vi "Close.vi"(8 "error in (no error)":errorcluster, 11 "reference in":refnum<class "Test_Sim.lvclass">) -> (0 "error out":errorcluster, 3 "reference in":refnum<class "Test_Sim.lvclass">)   [LabVIEW 2020, in "Test_Sim.lvlib" / "Test_Sim.lvclass"]
uses:
  Test_Sim.lvclass
  Components/Test_Base.lvlibp/Test_Base.lvclass
  Components/ViPER.lvlibp/ViPER.lvclass
  C:/Projects/Medulla/Presentations/Sydney_LVUG/Demo/Flux_Capacitor_Tester/Components/ViPER.lvlibp/ViPER.lvclass
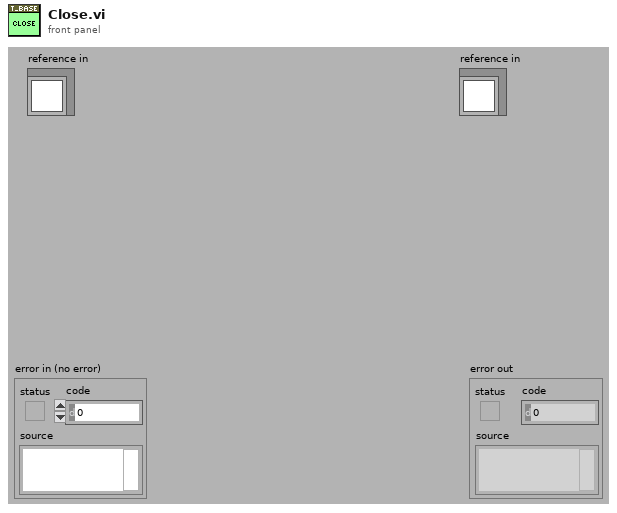
[diagram p1: front panel]
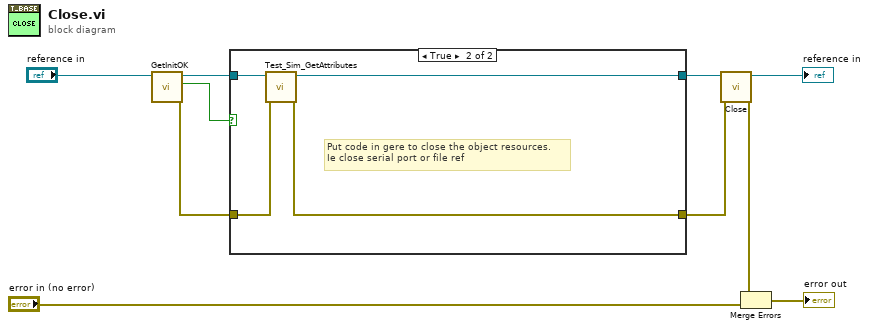
[diagram p0: block diagram]
diagram:
  n1 = call "GetInitOK.vi"("reference in"="reference in") -> ("error out"=w4:errorcluster, "init_ok"=w5:bool, "reference out"=w6:refnum<class "Test_Sim.lvclass">)  [unwired: 8 in]
  n2 = case shown="True" w5 {
    tunnel: w4 -> [w12 w15]
    tunnel: [w12 w14] -> w7
    tunnel: w6 -> [w11 w16]
    tunnel: [w11 w13] -> w8
    frame False {
    }
    frame True {
      # "Put code in gere to close the object resources.\nIe close serial port or file ref"
      n3 = call "Test_Sim_GetAttributes.vi"("error in (no error)"=w15, "reference in"=w16) -> ("error out"=w14:errorcluster, "reference out"=w13:refnum<class "Test_Sim.lvclass">)  [unwired: 6 in, 2 out]
    }
  }
  n4 = call-parent "Close.vi"("error in (no error)"=w7, "reference in"=w8) -> ("error out"=w3:errorcluster, "reference in"=→"reference in":refnum<class "Test_Sim.lvclass">)  [unwired: 8 in]
  n5 = Merge Errors(w3, "error in (no error)") -> (→"error out":errorcluster)
